vi "scan_generate_stage_positions.vi"(5 "travel_min (mm)":dbl, 7 "travel_max (mm)":dbl, 8 "error in (no error)":errorcluster, 10 "scan_position_settings":T1, 11 "scan_panel in":refnum<class "scan_panel.lvclass">) -> (0 "error out":errorcluster, 2 "Positions (mm)":dbl[](array[numeric]), 3 "scan_panel out":refnum<class "scan_panel.lvclass">)   [LabVIEW 2015, in "scan_panel.lvclass"]
uses:
  scan_panel.lvclass
  scan_position_settings.ctl
  scan_unit.ctl
  scan_panel.lvclass/scan_panel.ctl
  <vilib>/Analysis/1siggen.llb/Ramp Pattern by Samples.vi
  <vilib>/Analysis/NI_AALBase.lvlib
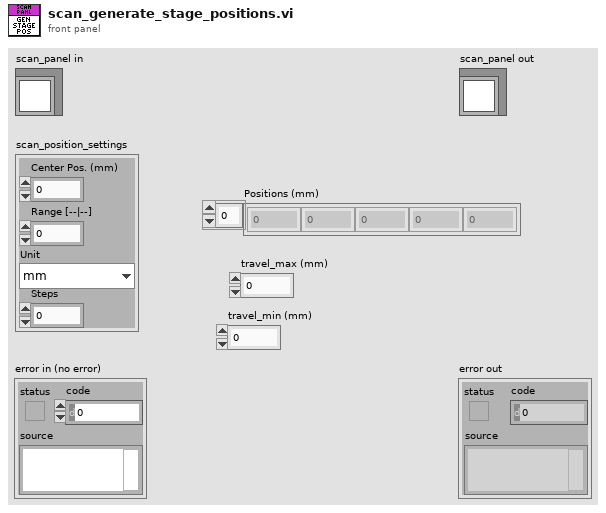
[diagram p1: front panel]
types:
  T1 = typedef "scan_position_settings.ctl" = cluster{"Center Pos. (mm)":dbl, "Range [--|--]":dbl, "Unit":T2, "Steps":dbl}
  T2 = typedef "scan_unit.ctl" = enum16{"mm", "s", "ms", "us", "ns", "ps", "fs"}
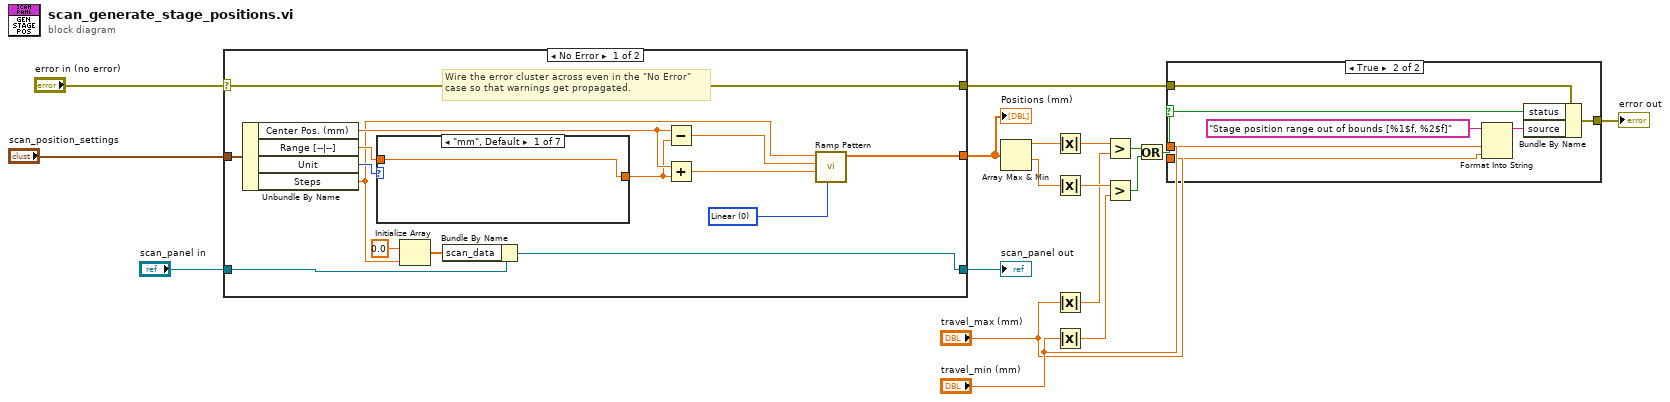
[diagram p0: block diagram]
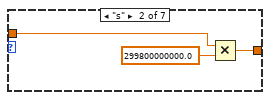
[diagram p3: hidden frame]
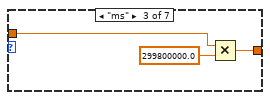
[diagram p4: hidden frame]
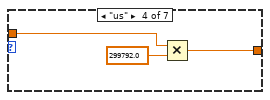
[diagram p5: hidden frame]
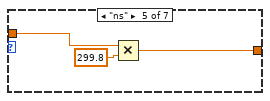
[diagram p6: hidden frame]
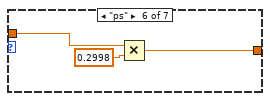
[diagram p7: hidden frame]
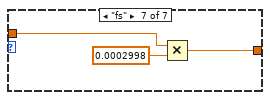
[diagram p8: hidden frame]
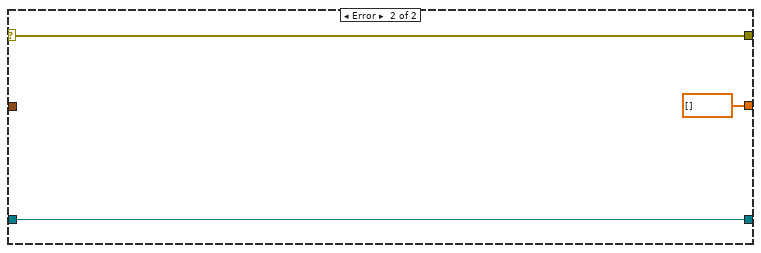
[diagram p9: hidden frame]
diagram:
  n1 = case shown="No Error" "error in (no error)" {
    selector: "error in (no error)" -> [w33 w55]
    tunnel: [w33 w55] -> w7
    tunnel: [w19 w54] -> w16
    tunnel: "scan_panel in" -> [w21 w54]
    tunnel: "scan_position_settings" -> [w32 _]
    tunnel: [w25 dbl[] [] ("Ramp Pattern")] -> w14
    frame No Error {
      w29 = u16 0 items=["Linear", "Logarithmic"] ("type")
      # "Wire the error cluster across even in the \"No Error\"\ncase so that warnings get propagated."
      n2 = Unbundle By Name(w32) -> ("Center Pos. (mm)"=w28:dbl, "Range [--|--]"=w30:dbl, "Unit"=w31:T2, "Steps"=w23:dbl)
      n3 = case shown="\"mm\", Default" w31 {
        tunnel: w30 -> [w34 w37 w38 w42 w44 w47 w50]
        tunnel: [w34 w35 w39 w41 w45 w48 w51] -> w24
        frame "mm", Default {
        }
        frame "s" {
          n4 = Multiply(x=w37, y=299800000000.0) -> (x*y=w35:dbl)
        }
        frame "ms" {
          n5 = Multiply(x=w38, y=299800000.0) -> (x*y=w39:dbl)
        }
        frame "us" {
          n6 = Multiply(x=w42, y=299792.0) -> (x*y=w41:dbl)
        }
        frame "ns" {
          n7 = Multiply(x=w44, y=299.8) -> (x*y=w45:dbl)
        }
        frame "ps" {
          n8 = Multiply(x=w47, y=0.2998) -> (x*y=w48:dbl)
        }
        frame "fs" {
          n9 = Multiply(x=w50, y=0.0002998) -> (x*y=w51:dbl)
        }
      }
      n10 = Initialize Array(0.0 ("element"), w23) -> (w20:dbl[])
      n11 = Bundle By Name(cluster=w21, "scan_data"=w20) -> (w19:refnum<class "scan_panel.lvclass">)
      n12 = Subtract(x=w28, y=w24) -> (x-y=w27:dbl)
      n13 = Add(x=w28, y=w24) -> (x+y=w26:dbl)
      n14 = call-poly <vilib>:"Ramp Pattern.vi"("type"=w29, "start"=w26, "end"=w27, "samples"=w23) -> ("Ramp Pattern"=w25:dbl[])  [unwired: 6 in, 1 out]
    }
    frame Error {
    }
  }
  "scan_panel out" <- w16
  "Positions (mm)" <- w14
  n15 = Array Max & Min(array=w14) -> (max value=w13:dbl, min value=w12:dbl)  [unwired: 2 out]
  n16 = Absolute Value(x=w13) -> (abs(x)=w11:dbl)
  n17 = Absolute Value(x=w12) -> (abs(x)=w10:dbl)
  n18 = Absolute Value(x="travel_max (mm)") -> (abs(x)=w3:dbl)
  n19 = Absolute Value(x="travel_min (mm)") -> (abs(x)=w4:dbl)
  n20 = Greater?(x=w11, y=w3) -> (0:w9:bool)
  n21 = Greater?(x=w10, y=w4) -> (0:w8:bool)
  n22 = Or(x=w9, y=w8) -> (x .or. y?=w6:bool)
  n23 = case shown="True" w6 {
    selector: w6 -> [_ w62]
    tunnel: w7 -> [w56 w63]
    tunnel: [w56 w61] -> w5
    tunnel: "travel_min (mm)" -> [_ w59]
    tunnel: "travel_max (mm)" -> [_ w58]
    frame False {
    }
    frame True {
      n24 = Format Into String(initial string="Stage position range out of bounds [%1$f, %2$f]" ("source"), w59, w58) -> (resulting string=w57:string)  [unwired: 2 in, 1 out]
      n25 = Bundle By Name(cluster=w63, "status"=w62, "source"=w57) -> (w61:errorcluster)
    }
  }
  "error out" <- w5
